vi "SwissSPAD Live_Control Label to Settings Element.vi"(2 "Control Label":string) -> (7 "Settings List Element":T1)   [LabVIEW 2021]
uses:
  SwissSPAD Live_Settings List.ctl
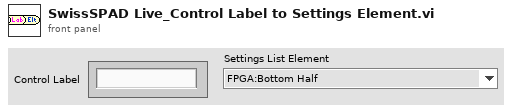
[diagram p1: front panel]
types:
  T1 = typedef "SwissSPAD Live_Settings List.ctl" = enum16{"FPGA:Bottom Half", "FPGA:Top Half", "FPGA:Bottom Bitfile Path", "FPGA:Top Bitfile Path", "FPGA:Bottom Bitstream Version", "FPGA:Top Bitstream Version", "FPGA:Auto Reset FPGA", "FPGA:Bottom FPGA Serial Number", "FPGA:Top FPGA Serial Number", "FPGA:Detector PCB Version", "Acquisition Parameters:Microlens", "Acquisition Parameters:SS2 DAQ Parameters", "Acquisition Parameters:Gate Configuration Array", "Acquisition Parameters:SS3 DAQ Parameters", "Acquisition Parameters:Buffer Size (# 8-bit Gates)", "File Information:File Information", "File Information:# Datasets in Series", "File Information:Scrambled File Flag", "File Information:SS3 Gate Slip Correction", "File Information:SS3 Hot Pixel Mismatch Detection", "File Information:Delay between Datasets", "File Information:Save Sum of All Gates Preview", "Image Parameters:Image ROI Information", "Image Parameters:Image Binning Options", "Image Parameters:SS3 Displayed Image", "Image Parameters:Image Display Options", "Image Parameters:Use Histogram Cursors", "Image Parameter:FPGA Data to Display", "UI Settings:Histogram Bins Number", "UI Settings:Use Image Display Options", "UI Settings:Verbose Settings", "UI Settings:Verbose Saving"}
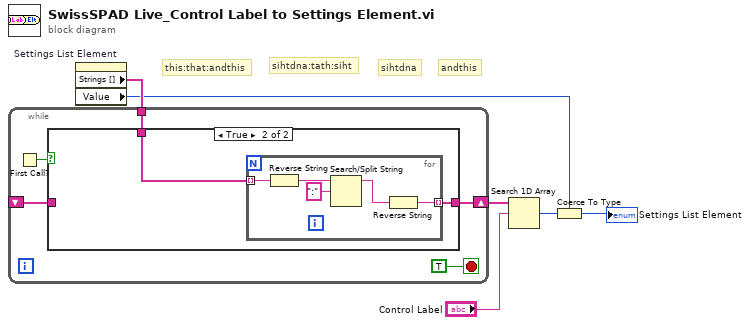
[diagram p0: block diagram]
diagram:
  # "andthis"
  # "sihtdna"
  # "sihtdna:tath:siht"
  # "this:that:andthis"
  n1 = property on="Settings List Element" class="Enum (strict)"() -> ("Strings []"=w2:string[], "Value"=w1:T1)  [unwired: 2 in, 2 out]
  n2 = while {
    shift-right: [w9] -> w6
    shift-left: _ -> [w8]
    tunnel: w2 -> [w7]
    stop <- TRUE stop-if-true
    n3 = First Call?() -> (First Call?: T/F=w10:bool)
    n4 = case shown="True" w10 {
      tunnel: [w12 w14] -> w9
      tunnel: w8 -> [w12 _]
      tunnel: w7 -> [_ w13]
      frame False {
      }
      frame True {
        n5 = for {
          tunnel: w13 -> [w19] mode=indexing
          tunnel: [w15] -> w14 mode=indexing
          n6 = Reverse String(1:w19) -> (0:w17:string)
          n7 = Search/Split String(string=w17, search string/char (-)=":") -> (substring before match=w16:string)  [unwired: 1 in, 2 out]
          n8 = Reverse String(1:w16) -> (0:w15:string)
        }
      }
    }
  }
  n9 = Search 1D Array(1D array=w6, element="Control Label") -> (index of element=w4:i32)  [unwired: 1 in]
  n10 = Coerce To Type(0:w4, 1:w1) -> (2:→"Settings List Element":T1)
